vi "FloatingPointStuff.vi"() -> ()   [LabVIEW 2016]
panel:
  in  "Y":sgl
  in  "X":sgl
  out "Z":sgl
  out "Output":u32 format="%0d"
  out "Y":u32=1112014848 format="%0d"
  out "X":u32=1112014848 format="%0d"
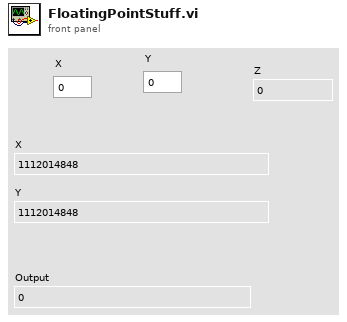
[diagram p1: front panel]
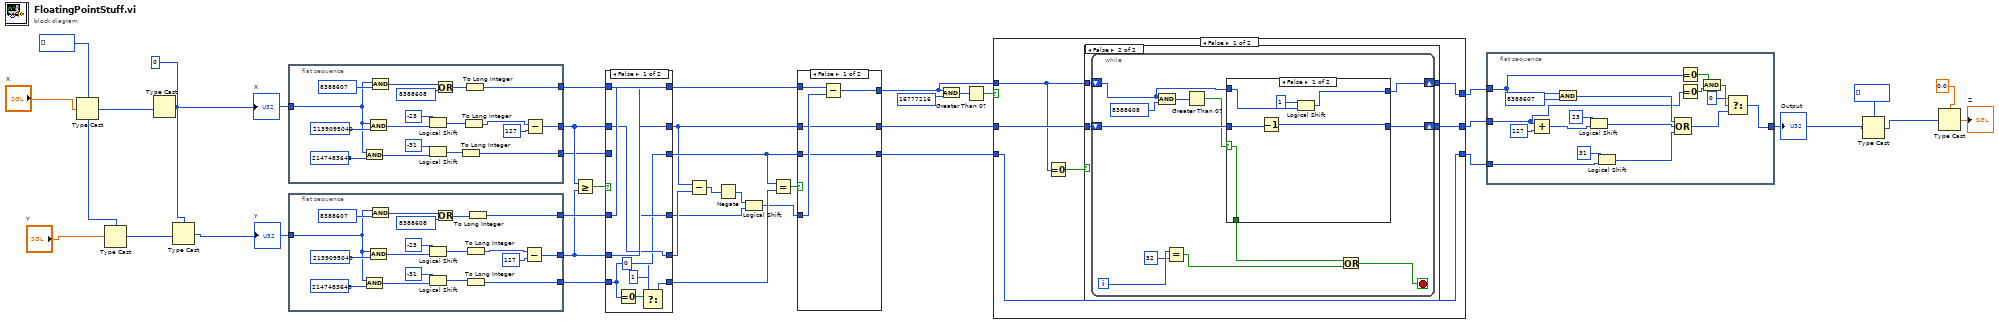
[diagram p0: block diagram]
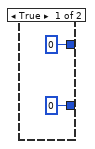
[diagram p3: hidden frame]
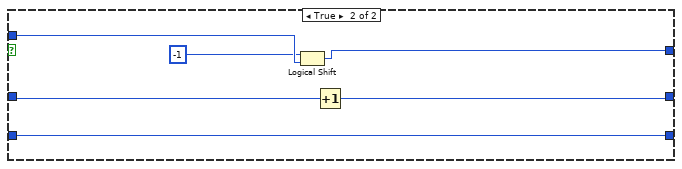
[diagram p5: hidden frame]
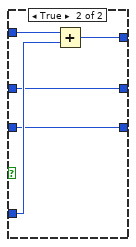
[diagram p6: hidden frame]
diagram:
  w3 = u32 0
  w4 = u8[] []
  n1 = Type Cast(type=w4, x="X") -> (*(type *) &x=w7:u8[])
  n2 = Type Cast(type=w4, x="Y") -> (*(type *) &x=w6:u8[])
  n3 = Type Cast(type=w3, x=w7) -> (*(type *) &x=w2:u32)
  "X" <- w2
  n4 = Type Cast(type=w3, x=w6) -> (*(type *) &x=w1:u32)
  "Y" <- w1
  n5 = flat-sequence {
    tunnel: w2 -> [w47]
    tunnel: [w46] -> w37
    tunnel: [w43] -> w38
    tunnel: [w40] -> w36
    frame #0 {
      n6 = And(x=w47, y=u32 2147483648) -> (x .and. y?=w49:u32)
      n7 = And(x=w47, y=u32 2139095040) -> (x .and. y?=w57:u32)
      n8 = And(x=w47, y=u32 8388607) -> (x .and. y?=w55:u32)
      n9 = Logical Shift(y=i16 -23, x=w57) -> (x << y=w45:u32)
      n10 = Logical Shift(y=i16 -31, x=w49) -> (x << y=w41:u32)
      n11 = Or(x=w55, y=u32 8388608) -> (x .or. y?=w44:u32)
      n12 = To Long Integer(number=w41) -> (32bit integer=w40:i32)
      n13 = To Long Integer(number=w45) -> (32bit integer=w42:i32)
      n14 = To Long Integer(number=w44) -> (32bit integer=w43:i32)
      n15 = Subtract(x=w42, y=127) -> (x-y=w46:i32)
    }
  }
  n16 = flat-sequence {
    tunnel: w1 -> [w65]
    tunnel: [w64] -> w34
    tunnel: [w59] -> w33
    tunnel: [w58] -> w35
    frame #0 {
      n17 = And(x=w65, y=u32 2147483648) -> (x .and. y?=w67:u32)
      n18 = And(x=w65, y=u32 2139095040) -> (x .and. y?=w75:u32)
      n19 = And(x=w65, y=u32 8388607) -> (x .and. y?=w73:u32)
      n20 = Logical Shift(y=i16 -23, x=w75) -> (x << y=w61:u32)
      n21 = Logical Shift(y=i16 -31, x=w67) -> (x << y=w62:u32)
      n22 = Or(x=w73, y=u32 8388608) -> (x .or. y?=w63:u32)
      n23 = To Long Integer(number=w61) -> (32bit integer=w60:i32)
      n24 = To Long Integer(number=w62) -> (32bit integer=w59:i32)
      n25 = To Long Integer(number=w63) -> (32bit integer=w58:i32)
      n26 = Subtract(x=w60, y=127) -> (x-y=w64:i32)
    }
  }
  n27 = Greater Or Equal?(x=w37, y=w34) -> (x >= y?=w39:bool)
  n28 = case shown="False" w39 {
    tunnel: w38 -> [w82 w90]
    tunnel: w37 -> [w81 w89]
    tunnel: w36 -> [_ w88]
    tunnel: w35 -> [w84 w87]
    tunnel: w34 -> [w83 w86]
    tunnel: w33 -> [w80 w85]
    tunnel: [w84 w90] -> w30
    tunnel: [w83 w89] -> w14
    tunnel: [w80 w88] -> w29
    tunnel: [w82 w87] -> w12
    tunnel: [w81 w86] -> w13
    tunnel: [w76 w85] -> w32
    frame False {
      n29 = Equal To 0?(x=w80) -> (x = 0?=w79:bool)
      n30 = Select(t=1 ("y"), s=w79, f=0) -> (s? t:f=w76:i32)
    }
    frame True {
    }
  }
  n31 = Subtract(x=w14, y=w13) -> (x-y=w11:i32)
  n32 = Negate(x=w11) -> (-x=w10:i32)
  n33 = Logical Shift(y=w10, x=w12) -> (x << y=w9:i32)
  n34 = Equal?(x=w29, y=w32) -> (x = y?=w31:bool)
  n35 = case shown="False" w31 {
    tunnel: w30 -> [w94 w99]
    tunnel: w9 -> [w95 w100]
    tunnel: [w92 w98] -> w23
    tunnel: w29 -> [w92 w98]
    tunnel: [w93 w97] -> w24
    tunnel: [w91 w96] -> w25
    tunnel: w14 -> [w91 w96]
    frame False {
      n36 = Subtract(x=w94, y=w95) -> (x-y=w93:i32)
    }
    frame True {
      n37 = Add(x=w99, y=w100) -> (x+y=w97:i32)
    }
  }
  n38 = And(x=w24, y=16777216) -> (x .and. y?=w27:i32)
  n39 = Greater Than 0?(x=w27) -> (x > 0?=w26:bool)
  n40 = case shown="False" w26 {
    tunnel: w25 -> [w106 w135]
    tunnel: w24 -> [w101 w138]
    tunnel: [w104 w134] -> w22
    tunnel: w23 -> [w105 w139]
    tunnel: [w105 w139] -> w21
    tunnel: [w103 w136] -> w20
    frame False {
      n41 = Equal To 0?(x=w101) -> (x = 0?=w102:bool)
      n42 = case shown="False" w102 {
        tunnel: w101 -> [_ w112]
        tunnel: w106 -> [_ w111]
        tunnel: [0 w110] -> w104
        tunnel: [0 w109] -> w103
        frame True {
        }
        frame False {
          n43 = while {
            shift-right: [w121] -> w109
            shift-left: w112 -> [w119]
            shift-right: [w120] -> w110
            shift-left: w111 -> [w122]
            i -> [w116]
            stop <- w113 stop-if-true
            n44 = And(x=w119, y=8388608) -> (x .and. y?=w123:i32)
            n45 = Equal?(x=w116, y=32) -> (x = y?=w114:bool)
            n46 = Greater Than 0?(x=w123) -> (x > 0?=w118:bool)
            n47 = case shown="False" w118 {
              selector: w118 -> [w130 w131]
              tunnel: w119 -> [w127 w133]
              tunnel: w122 -> [w129 w132]
              tunnel: [w125 w133] -> w121
              tunnel: [w128 w132] -> w120
              tunnel: [w130 w131] -> w117
              frame False {
                n48 = Decrement(x=w129) -> (x-1=w128:i32)
                n49 = Logical Shift(y=i16 1, x=w127) -> (x << y=w125:i32)
              }
              frame True {
              }
            }
            n50 = Or(x=w117, y=w114) -> (x .or. y?=w113:bool)
          }
        }
      }
    }
    frame True {
      n51 = Logical Shift(y=i16 -1, x=w138) -> (x << y=w136:i32)
      n52 = Increment(x=w135) -> (x+1=w134:i32)
    }
  }
  n53 = flat-sequence {
    tunnel: w22 -> [w141]
    tunnel: w21 -> [w152]
    tunnel: w20 -> [w140]
    tunnel: [w146] -> w15
    frame #0 {
      n54 = Add(x=w141, y=127) -> (x+y=w154:i32)
      n55 = And(x=w140, y=u32 8388607) -> (x .and. y?=w148:u32)
      n56 = Logical Shift(y=i16 23, x=w154) -> (x << y=w149:i32)
      n57 = Logical Shift(y=i16 31, x=w152) -> (x << y=w150:i32)
      n58 = Compound Arithmetic op=OR(w148, w149, w150) -> (w147:u32)
      n59 = Equal To 0?(x=w140) -> (x = 0?=w145:bool)
      n60 = Equal To 0?(x=w141) -> (x = 0?=w144:bool)
      n61 = And(x=w145, y=w144) -> (x .and. y?=w143:bool)
      n62 = Select(t=u32 0, s=w143, f=w147) -> (s? t:f=w146:u32)
    }
  }
  n63 = Type Cast(type=u8[] [], x=w15) -> (*(type *) &x=w17:u8[])
  n64 = Type Cast(type=sgl 0.0, x=w17) -> (*(type *) &x=→"Z":sgl)
  "Output" <- w15
